vi "AddonMotors Check for New Command.vi"(9 "Current Command":T14={"Default Command"={"Operation"=enum."Reserve", "Setpoint"=0.0, "Duration"=0.0, "Motor Ref"={"MotorRef"={"DeviceStatus"={"status"=FALSE, "code"=20, "source"=""}, "Type"=enum."PWM", "PWM"={"PWM Channel"=enum."PWM 0", "DeadBand"={"Name"="", "maxPositivePwm"=0, "minPositivePwm"=0, "centerPwm"=0, "maxNegativePwm"=0, "minNegativePwm"=0, "angularRange"=0}}, "CAN"={"Device Number"=0, "Control Mode"=enum."Voltage", "Semaphore"=refnum, "Max Vout"=0.0, "TalonSRX Control Mode"=enum."Percent VBus"}, "Invert"=FALSE}, "Encoder Ticks Per Rev"=0.0, "Set Position"=0.0}}, "Command Timing"={"Start Time (ms)"=0, "Iterations"=0}, "Command Arguments"={"Command Info"={"Name"="", "Status"=enum."Successful", "notifier out"=refnum}, "Description"="", "Default Command"={"Operation"=enum."Reserve", "Setpoint"=0.0, "Duration"=0.0, "Motor Ref"={"MotorRef"={"DeviceStatus"={"status"=FALSE, "code"=20, "source"=""}, "Type"=enum."PWM", "PWM"={"PWM Channel"=enum."PWM 0", "DeadBand"={"Name"="", "maxPositivePwm"=0, "minPositivePwm"=0, "centerPwm"=0, "maxNegativePwm"=0, "minNegativePwm"=0, "angularRange"=0}}, "CAN"={"Device Number"=0, "Control Mode"=enum."Voltage", "Semaphore"=refnum, "Max Vout"=0.0, "TalonSRX Control Mode"=enum."Percent VBus"}, "Invert"=FALSE}, "Encoder Ticks Per Rev"=0.0, "Set Position"=0.0}}, "notifier out"=refnum, "Subsystem Name"=""}}, 10 "Wait time (ms)":dbl, 11 "Finished?":bool) -> (0 "Completion":T12, 1 "Subsystem Name":string, 2 "Current Command":T1={"Operation"=enum."Reserve", "Setpoint"=0.0, "Duration"=0.0, "Motor Ref"={"MotorRef"={"DeviceStatus"={"status"=FALSE, "code"=20, "source"=""}, "Type"=enum."PWM", "PWM"={"PWM Channel"=enum."PWM 0", "DeadBand"={"Name"="", "maxPositivePwm"=0, "minPositivePwm"=0, "centerPwm"=0, "maxNegativePwm"=0, "minNegativePwm"=0, "angularRange"=0}}, "CAN"={"Device Number"=0, "Control Mode"=enum."Voltage", "Semaphore"=refnum, "Max Vout"=0.0, "TalonSRX Control Mode"=enum."Percent VBus"}, "Invert"=FALSE}, "Encoder Ticks Per Rev"=0.0, "Set Position"=0.0}}, 3 "Initial Trace String":string, 4 "NextCommand":T14={"Default Command"={"Operation"=enum."Reserve", "Setpoint"=0.0, "Duration"=0.0, "Motor Ref"={"MotorRef"={"DeviceStatus"={"status"=FALSE, "code"=20, "source"=""}, "Type"=enum."PWM", "PWM"={"PWM Channel"=enum."PWM 0", "DeadBand"={"Name"="", "maxPositivePwm"=0, "minPositivePwm"=0, "centerPwm"=0, "maxNegativePwm"=0, "minNegativePwm"=0, "angularRange"=0}}, "CAN"={"Device Number"=0, "Control Mode"=enum."Voltage", "Semaphore"=refnum, "Max Vout"=0.0, "TalonSRX Control Mode"=enum."Percent VBus"}, "Invert"=FALSE}, "Encoder Ticks Per Rev"=0.0, "Set Position"=0.0}}, "Command Timing"={"Start Time (ms)"=0, "Iterations"=0}, "Command Arguments"={"Command Info"={"Name"="", "Status"=enum."Successful", "notifier out"=refnum}, "Description"="", "Default Command"={"Operation"=enum."Reserve", "Setpoint"=0.0, "Duration"=0.0, "Motor Ref"={"MotorRef"={"DeviceStatus"={"status"=FALSE, "code"=20, "source"=""}, "Type"=enum."PWM", "PWM"={"PWM Channel"=enum."PWM 0", "DeadBand"={"Name"="", "maxPositivePwm"=0, "minPositivePwm"=0, "centerPwm"=0, "maxNegativePwm"=0, "minNegativePwm"=0, "angularRange"=0}}, "CAN"={"Device Number"=0, "Control Mode"=enum."Voltage", "Semaphore"=refnum, "Max Vout"=0.0, "TalonSRX Control Mode"=enum."Percent VBus"}, "Invert"=FALSE}, "Encoder Ticks Per Rev"=0.0, "Set Position"=0.0}}, "notifier out"=refnum, "Subsystem Name"=""}})   [LabVIEW 2015]
uses:
  AddonMotors Setpoints.ctl
  AddonMotors Operations.ctl
  Framework/Detailed Motor Type Def.ctl
  <vilib>/Rock Robotics/WPI/MotorControl/WPI_MotorControlDeviceRef.ctl
  <vilib>/Rock Robotics/WPI/MotorControl/WPI_MotorControlType.ctl
  <vilib>/Rock Robotics/SystemInterfaces/DIO/FPGA_DIOPWMChannel.ctl
  <vilib>/Rock Robotics/WPI/PWM/WPI_PWMDeadband.ctl
  <vilib>/Rock Robotics/WPI/CAN/Jaguar/SubVIs/WPI_CANJaguar_ControlMode.ctl
  <vilib>/Rock Robotics/WPI/CAN/TalonSRX/WPI_CANTalonSRX_APIControlMode.ctl
  <vilib>/Rock Robotics/WPI/Framework/Command Status Info.ctl
  <vilib>/Rock Robotics/WPI/Framework/Completion Status.ctl
  <vilib>/Rock Robotics/WPI/Framework/Completion Notifier.ctl
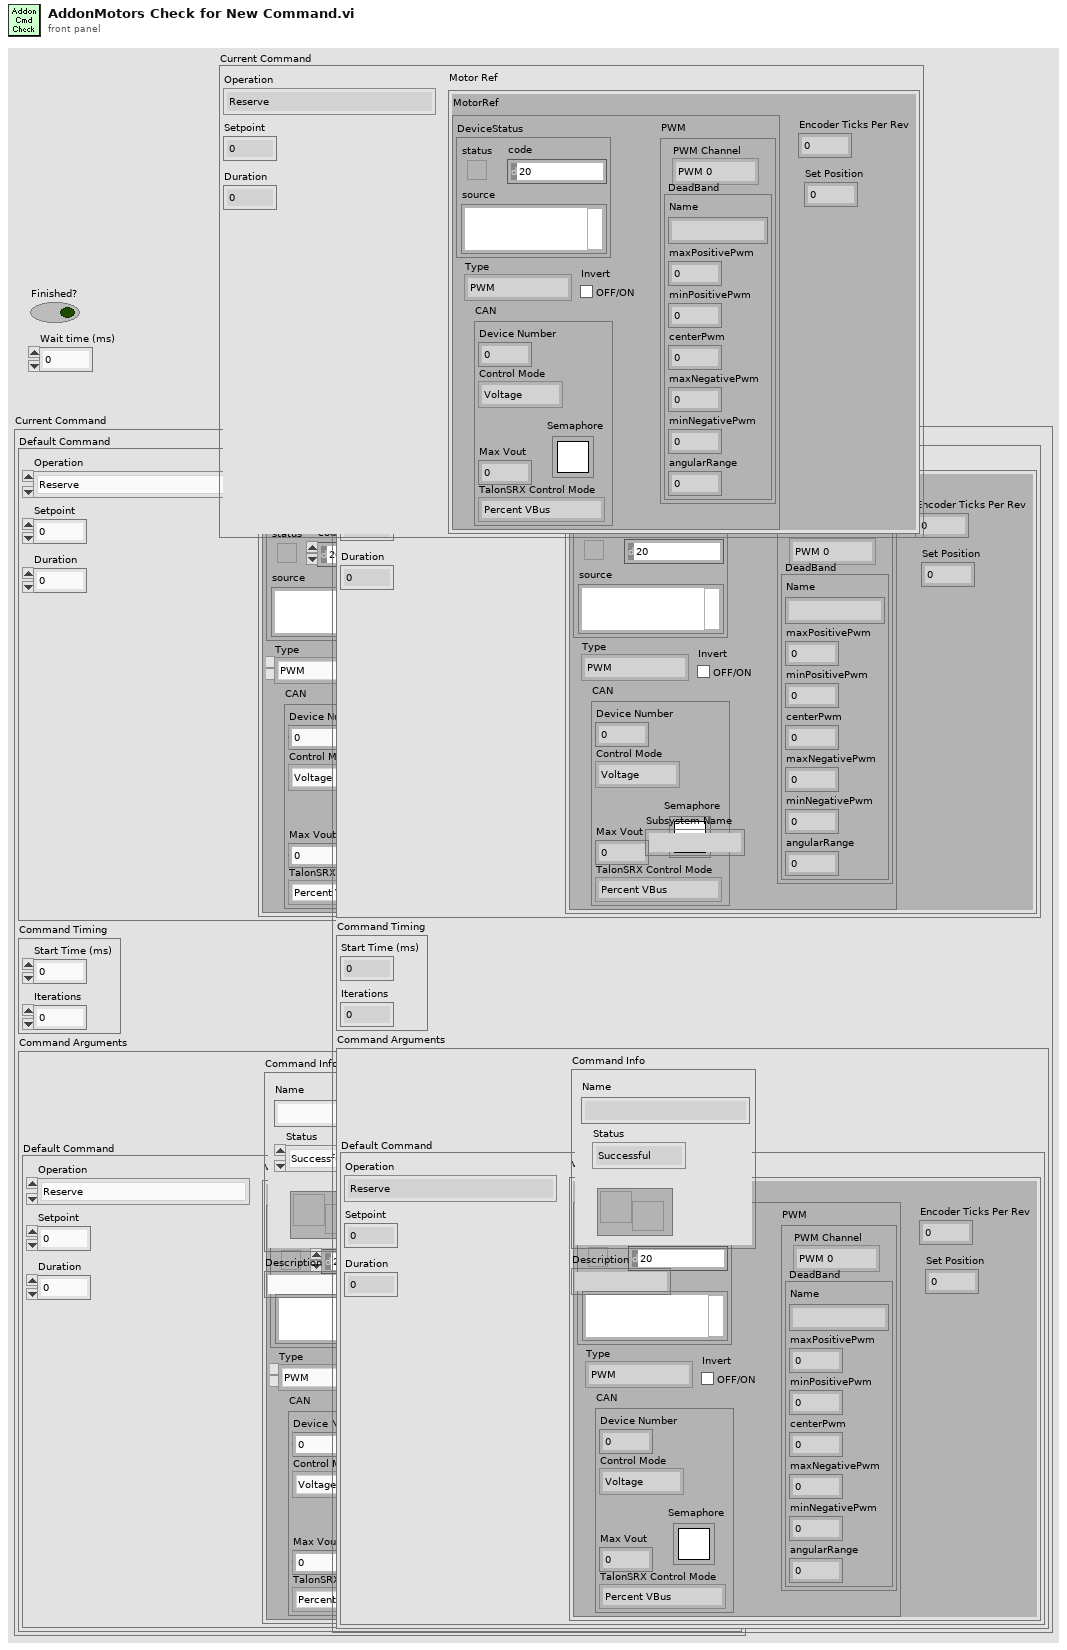
[diagram p1: front panel]
types:
  T1 = typedef "AddonMotors Setpoints.ctl" = cluster{"Operation":T2, "Setpoint":dbl, "Duration":dbl, "Motor Ref":T3}
  T2 = typedef "AddonMotors Operations.ctl" = enum16{"Reserve", "Read Current", "Immediate", "Angle (Position)", "Speed", "Angle Increments (Position)"}
  T3 = typedef "Detailed Motor Type Def.ctl" = cluster{"MotorRef":T4, "Encoder Ticks Per Rev":dbl, "Set Position":dbl}
  T4 = typedef "WPI_MotorControlDeviceRef.ctl" = cluster{"DeviceStatus":errorcluster, "Type":T5, "PWM":cluster{"PWM Channel":T6, "DeadBand":T7}, "CAN":cluster{"Device Number":u8, "Control Mode":T8, "Semaphore":T9, "Max Vout":dbl, "TalonSRX Control Mode":T10}, "Invert":bool}
  T5 = typedef "WPI_MotorControlType.ctl" = enum16{"PWM", "CAN", "CANTalonSRX"}
  T6 = typedef "FPGA_DIOPWMChannel.ctl" = enum8{"PWM 0", "PWM 1", "PWM 2", "PWM 3", "PWM 4", "PWM 5", "PWM 6", "PWM 7", "PWM 8", "PWM 9", "PWM MXP 0", "PWM MXP 1", "PWM MXP 2", "PWM MXP 3", "PWM MXP 4", "PWM MXP 5", "PWM MXP 6", "PWM MXP 7", "PWM MXP 8", "PWM MXP 9", "Invalid"}
  T7 = typedef "WPI_PWMDeadband.ctl" = cluster{"Name":string, "maxPositivePwm":i32, "minPositivePwm":i32, "centerPwm":i32, "maxNegativePwm":i32, "minNegativePwm":i32, "angularRange":u16}
  T8 = typedef "WPI_CANJaguar_ControlMode.ctl" = enum8{"Percent VBus", "Current", "Speed", "Position", "Voltage"}
  T9 = typedef "Semaphore RefNum" = refnum<k1>
  T10 = typedef "WPI_CANTalonSRX_APIControlMode.ctl" = enum8{"Percent VBus", "Speed", "Position", "Slave", "Unchanged / Invalid", "Voltage Compensation", "Current", "Motion Profile"}
  T11 = typedef "Command Status Info.ctl" = cluster{"Name":string, "Status":T12, "notifier out":T13}
  T12 = typedef "Completion Status.ctl" = enum16{"Successful", "Aborted", "Incomplete"}
  T13 = typedef "Completion Notifier.ctl" = refnum<notifier>
  T14 = cluster{"Default Command":T1, "Command Timing":cluster{"Start Time (ms)":u32, "Iterations":i32}, "Command Arguments":cluster{"Command Info":T11, "Description":string, "Default Command":T1, "notifier out":refnum<notifier>, "Subsystem Name":string}}
  T15 = cluster{"Command Info":T11, "Description":string, "Default Command":T1, "notifier out":refnum<notifier>, "Subsystem Name":string}
  T16 = cluster{"Default Command":T1, "Command Info":T11, "Description":string}
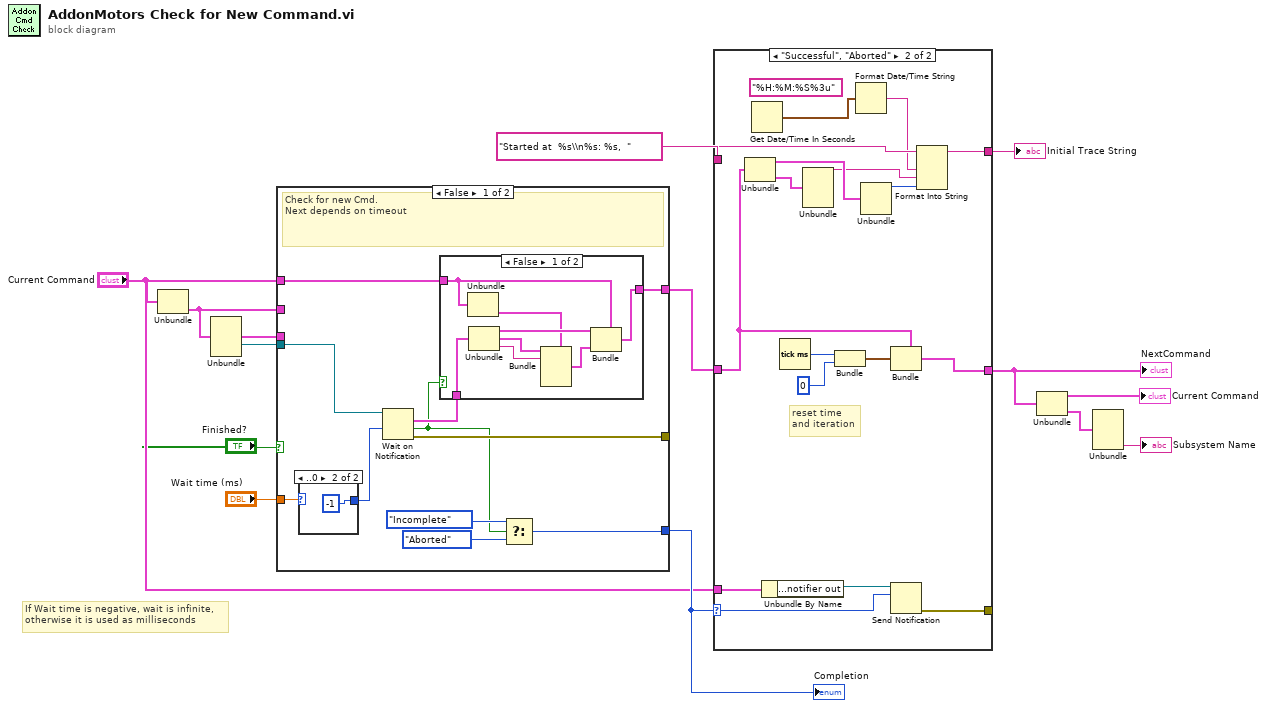
[diagram p0: block diagram]
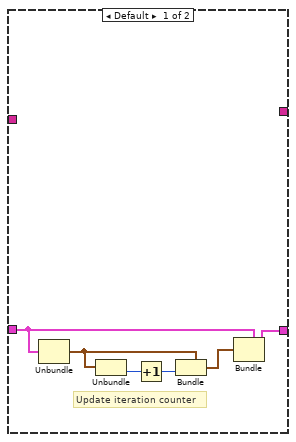
[diagram p2: hidden frame]
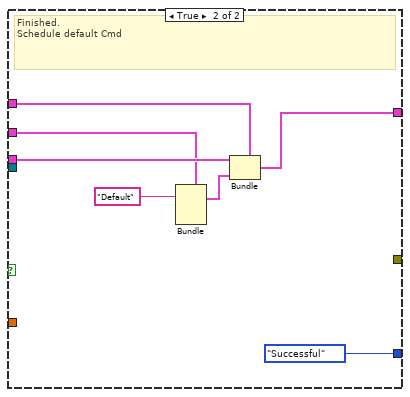
[diagram p5: hidden frame]
diagram:
  # "If Wait time is negative, wait is infinite,\notherwise it is used as milliseconds"
  n1 = Unbundle("Current Command") -> ("Command Arguments"=w1:T15)  [unwired: 2 out]
  n2 = Unbundle(w1) -> ("Default Command"=w4:T1, "notifier out"=w5:refnum<notifier>)  [unwired: 3 out]
  n3 = case shown="False" "Finished?" {
    tunnel: [w15 w42] -> w10
    tunnel: "Wait time (ms)" -> [w20 _]
    tunnel: [w23 Completion_Status."Successful"] -> w14
    tunnel: [w25 _] -> _
    tunnel: w5 -> [w24 _]
    tunnel: "Current Command" -> [w17 w41]
    tunnel: w4 -> [_ w40]
    tunnel: w1 -> [_ w38]
    frame False {
      # "Check for new Cmd.\nNext depends on timeout"
      n4 = case shown="..0" w20 {
        selector: w20 -> [w35 _]
        tunnel: [w35 -1] -> w19
        frame Default {
        }
        frame ..0 {
        }
      }
      n5 = Wait on Notification(notifier=w24, timeout in ms (-1)=w19) -> (notification=w18:T16, timed out?=w16:bool, error out=w25:errorcluster)  [unwired: 2 in, 1 out]
      n6 = case shown="False" w16 {
        tunnel: w18 -> [w33 _]
        tunnel: w17 -> [w30 w34]
        tunnel: [w26 w34] -> w15
        frame False {
          n7 = Unbundle(w30) -> ("Command Arguments"=w29:T15)  [unwired: 2 out]
          n8 = Unbundle(w33) -> ("Default Command"=w32:T1, "Command Info"=w27:T11, "Description"=w28:string)
          n9 = Bundle(cluster=w29, "Command Info"=w27, "Description"=w28) -> (w31:T15)  [unwired: 3 in]
          n10 = Bundle(cluster=w30, "Default Command"=w32, "Command Arguments"=w31) -> (w26:T14)  [unwired: 1 in]
        }
        frame True {
        }
      }
      n11 = Select(t=Completion_Status."Incomplete", s=w16, f=Completion_Status."Aborted") -> (s? t:f=w23:T12)
    }
    frame True {
      # "Finished.\nSchedule default Cmd"
      n12 = Bundle(cluster=w38, "Description"="Default") -> (w39:T15)  [unwired: 4 in]
      n13 = Bundle(cluster=w41, "Default Command"=w40, "Command Arguments"=w39) -> (w42:T14)  [unwired: 1 in]
    }
  }
  "Completion" <- w14
  n14 = case shown="\"Successful\", \"Aborted\"" w14 {
    selector: w14 -> [_ w66]
    tunnel: "Current Command" -> [_ w63]
    tunnel: "Started at  %s\\n%s: %s,  " ("format string") -> [_ w62]
    tunnel: [_ w61] -> w12
    tunnel: w10 -> [w46 w50]
    tunnel: [w47 w57] -> w9
    tunnel: [_ w54] -> _
    frame Default {
      # "Update iteration counter"
      n15 = Unbundle(w46) -> ("Command Timing"=w45:cluster{"Start Time (ms)":u32, "Iterations":i32})  [unwired: 2 out]
      n16 = Unbundle(w45) -> ("Iterations"=w48:i32)  [unwired: 1 out]
      n17 = Increment(x=w48) -> (x+1=w49:i32)
      n18 = Bundle(cluster=w45, "Iterations"=w49) -> (w44:cluster{"Start Time (ms)":u32, "Iterations":i32})  [unwired: 1 in]
      n19 = Bundle(cluster=w46, "Command Timing"=w44) -> (w47:T14)  [unwired: 2 in]
    }
    frame "Successful", "Aborted" {
      (unwired) "%H:%M:%S%3u" ("time format string (%c)")
      # "reset time\nand iteration"
      n20 = Unbundle(w50) -> ("Default Command"=w60:T1, "Command Arguments"=w55:T15)  [unwired: 1 out]
      n21 = Get Date/Time In Seconds() -> (seconds since 1Jan1904=w53:timestamp)
      n22 = Unbundle By Name(w63) -> ("Command Arguments.Command Info.notifier out"=w65:T13)
      n23 = Tick Count (ms)() -> (millisecond timer value=w59:u32)
      n24 = Unbundle(w55) -> ("Description"=w52:string)  [unwired: 4 out]
      n25 = Bundle("millisecond timer value"=w59, 0) -> (w56:cluster{"millisecond timer value":u32, i32})  [unwired: 1 in]
      n26 = Format Date/Time String(seconds (now)=w53) -> (date/time string=w51:string)  [unwired: 2 in]
      n27 = Unbundle(w60) -> ("Operation"=w64:T2)  [unwired: 3 out]
      n28 = Bundle(cluster=w50, "Command Timing"=w56) -> (w57:T14)  [unwired: 2 in]
      n29 = Send Notification(notification=w66, notifier=w65) -> (error out=w54:errorcluster)  [unwired: 1 in, 1 out]
      n30 = Format Into String(format string=w62, w51, w52, w64) -> (resulting string=w61:string)  [unwired: 2 in, 1 out]
    }
  }
  "NextCommand" <- w9
  "Initial Trace String" <- w12
  n31 = Unbundle(w9) -> ("Default Command"=→"Current Command":T1, "Command Arguments"=w3:T15)  [unwired: 1 out]
  n32 = Unbundle(w3) -> ("Subsystem Name"=→"Subsystem Name":string)  [unwired: 4 out]
